vi "Waveform Attribute, Get DBL Reference Array.vi"(5 "refnum array":refnum<vi>[](array[refnum]), 6 "error in":errorcluster, 9 "waveform":waveform(dbl)) -> (0 "error out":errorcluster, 1 "found":bool[](array[boolean]), 2 "values":dbl[](array[numeric]), 3 "waveform dup":waveform(dbl), 4 "found all values":bool)   [LabVIEW 2010]
doc: "Reads an array of Digital double precision (DBL) values from the waveform attributes using control references."
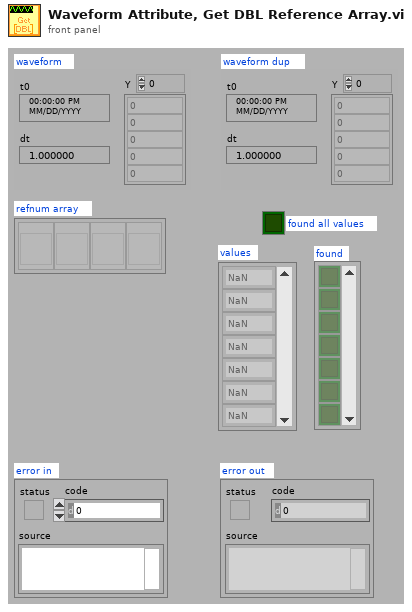
[diagram p1: front panel]
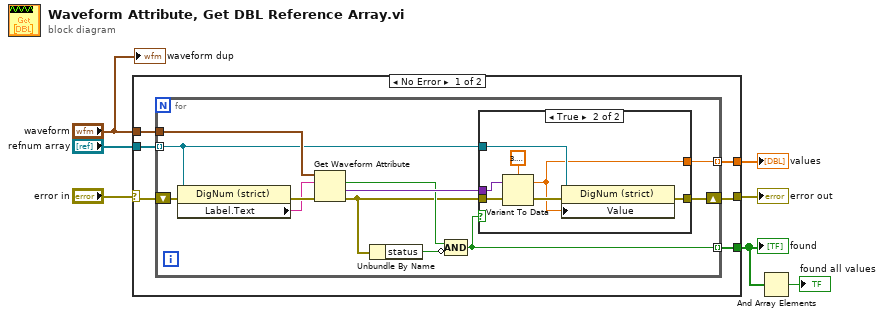
[diagram p0: block diagram]
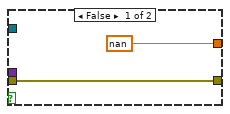
[diagram p2: hidden frame]
diagram:
  n1 = case shown="No Error" "error in" {
    selector: "error in" -> [w11 w35]
    tunnel: [w12 w35] -> w7
    tunnel: "waveform" -> [w10 _]
    tunnel: "refnum array" -> [w13 _]
    tunnel: [w9 _] -> w3
    tunnel: [w8 _] -> w1
    frame No Error {
      n2 = for {
        tunnel: w13 -> [w20] mode=indexing
        shift-right: [w21] -> w12
        shift-left: w11 -> [w25]
        tunnel: w10 -> [w24]
        tunnel: [w18] -> w9 mode=indexing
        tunnel: [w14] -> w8 mode=indexing
        n3 = property class="DigNum (strict)"(reference=w20, error in=w25) -> (error out=w23:errorcluster, "Label.Text"=w22:string)  [unwired: 1 out]
        n4 = Get Waveform Attribute(4:w23, 6:w22, 7:w24) -> (0:w15:errorcluster, 1:w19:variant, 2:w17:bool)  [unwired: 1 in, 1 out]
        n5 = Unbundle By Name(w15) -> ("status"=w16:bool)
        n6 = Compound Arithmetic op=AND(w17, invert w16) -> (w14:bool)
        n7 = case shown="True" w14 {
          tunnel: [w26 w34] -> w21
          tunnel: w20 -> [_ w33]
          tunnel: w19 -> [_ w32]
          tunnel: w15 -> [w26 w29]
          tunnel: [nan w28] -> w18
          frame False {
          }
          frame True {
            n8 = Variant To Data(error in=w29, Variant=w32, type=3.141592653589793) -> (error out=w30:errorcluster, data=w28:dbl)
            n9 = property class="DigNum (strict)"(reference=w33, error in=w30, "Value"=w28) -> (error out=w34:errorcluster)  [unwired: 1 out]
          }
        }
      }
    }
    frame Error {
    }
  }
  "error out" <- w7
  "found" <- w1
  "values" <- w3
  n10 = And Array Elements(Boolean array=w1) -> (logical AND=→"found all values":bool)
  "waveform dup" <- "waveform"
